vi "Lifetime at UC Intersection (gated).vi"(8 "Error In":errorcluster, 11 "Data for Pseudo UC Intersections":T1={"Linear Coefficients"={"u"=0.0, "v"=0.0}, "Decay Definition"={"offset: t0"=0.0, "period: T"=0.0, "lifetime: tau"=0.0, "Incident Signal: I"=0.0, "Normalized Decays"=FALSE, "IRF Model"=enum."Dirac", "IRF Parameter 1"=0.0, "Poisson Signal"=FALSE}, "Gates Definitions"={"First Gate: t1"=0.0, "Gate Width: W"=0.0, "Gate Step: d"=0.0, "# Gates: G"=0.0, "Use Gate Center"=FALSE, "Frames/Image: F"=0, "Gates/Frame: L"=0, "Bits/Frame: q"=0, "Multiplicity: p"=0, "Gate Type"=enum."Square", "Gate Edge s"=4.0, "Gate Top Slope"=4.0, "Reversed Sawtooth?"=FALSE, "Computation"=FALSE, "User-defined Gate"={"X Array"=[], "Y Array"=[]}, "Tolerance"=50.0, "Integration"=enum."Item 0", "# Steps"=50.0, "Type of User-defined Function"=enum."Gate"}, "iw"=0.0+0.0i, "Phasor Calculation"=enum."Direct Sum"}) -> (0 "Error Out":errorcluster, 1 "Analytical Solution 1":dbl[unit], 3 "Analytical Solution 2":dbl[unit])   [LabVIEW 2019]
uses:
  Data for SEPL Intersections.ctl
  Decay Definiton.ctl
  IRF Model.ctl
  Gate Definitions.ctl
  Gate Type.ctl
  Graphs/XY Graph/XY Plot Data.ctl
  Phasor Calculation Type.ctl
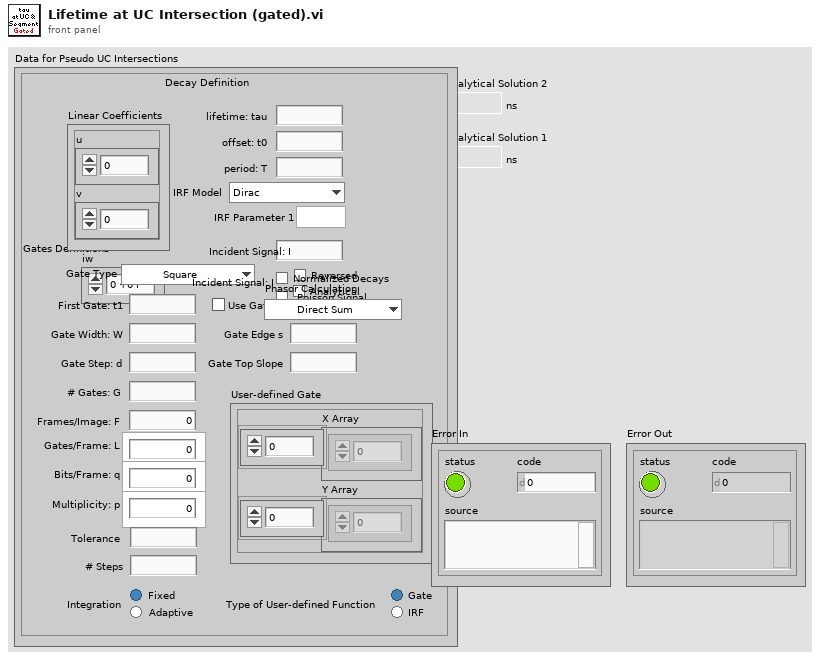
[diagram p1: front panel]
types:
  T1 = typedef "Data for SEPL Intersections.ctl" = cluster{"Linear Coefficients":cluster{"u":dbl, "v":dbl}, "Decay Definition":T2, "Gates Definitions":T4, "iw":cdb, "Phasor Calculation":T7}
  T2 = typedef "Decay Definiton.ctl" = cluster{"offset: t0":ext, "period: T":ext, "lifetime: tau":ext, "Incident Signal: I":ext, "Normalized Decays":bool, "IRF Model":T3, "IRF Parameter 1":ext, "Poisson Signal":bool}
  T3 = typedef "IRF Model.ctl" = enum16{"Dirac", "Exponential"}
  T4 = typedef "Gate Definitions.ctl" = cluster{"First Gate: t1":ext, "Gate Width: W":ext, "Gate Step: d":ext, "# Gates: G":ext, "Use Gate Center":bool, "Frames/Image: F":i32, "Gates/Frame: L":i32, "Bits/Frame: q":i32, "Multiplicity: p":i32, "Gate Type":T5, "Gate Edge s":ext, "Gate Top Slope":ext, "Reversed Sawtooth?":bool, "Computation":bool, "User-defined Gate":T6, "Tolerance":ext, "Integration":enum32{"Item 0", "Item 1"}, "# Steps":ext, "Type of User-defined Function":enum32{"Gate", "IRF"}}
  T5 = typedef "Gate Type.ctl" = enum16{"Square", "Finite Edge Square", "Finite Edge, Tilted Top Square", "Triangle", "Sawtooth", "User-defined"}
  T6 = typedef "XY Plot Data.ctl" = cluster{"X Array":dbl[], "Y Array":dbl[]}
  T7 = typedef "Phasor Calculation Type.ctl" = enum16{"Direct Sum", "Analytical Formula"}
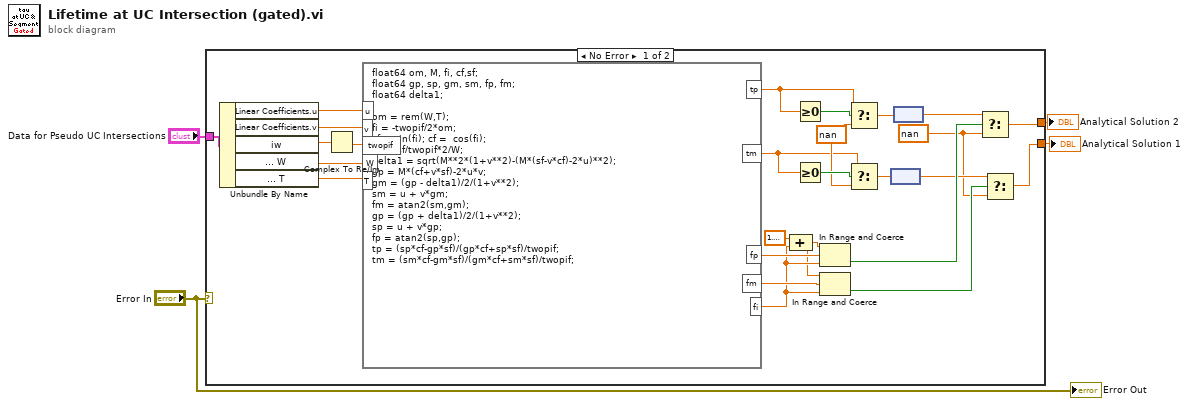
[diagram p0: block diagram]
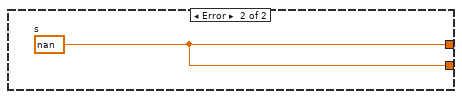
[diagram p2: hidden frame]
diagram:
  n1 = case shown="No Error" "Error In" {
    tunnel: "Data for Pseudo UC Intersections" -> [w30 _]
    tunnel: [w13 w31] -> w3
    tunnel: [w19 w31] -> w2
    frame No Error {
      w6 = nan ("f")
      w12 = dbl[unit] nan ("f")
      n2 = Unbundle By Name(w30) -> ("Linear Coefficients.u"=w29:dbl, "Linear Coefficients.v"=w28:dbl, "iw"=w27:cdb, "Gates Definitions.Gate Width: W"=w25:ext, "Decay Definition.period: T"=w24:ext)
      n3 = Complex To Re/Im(x + iy=w27) -> (y=w26:dbl)  [unwired: 1 out]
      n4 = formula code="float64 om, M, fi, cf,sf;\nfloat64 gp, sp, gm, sm, fp, fm;\nfloat64 delta1;\n\nom = rem(W,T);\nfi = -twopif/2*om;\nsf = sin(fi); cf =  cos(fi);\nM = -sf/twopif*2/W;\ndelta1 = sqrt(M**2*(1+v**2)-(M*(sf-v*cf)-2*u)**2);\ngp = M*(cf+v*sf)-2*u*v;\ngm = (gp - delta1)/2/(1+v**2);\nsm = u + v*gm;\nfm = atan2(sm,gm);\ngp = (gp + delta1)/2/(1+v**2);\nsp = u + v*gp;\nfp = atan2(sp,gp); \ntp = (sp*cf-gp*sf)/(gp*cf+sp*sf)/twopif;\ntm = (sm*cf-gm*sf)/(gm*cf+sm*sf)/twopif;"("u"=w29, "v"=w28, "twopif"=w26, "W"=w25, "T"=w24) -> ("tm"=w5:dbl, "tp"=w10:dbl, "fp"=w23:dbl, "fm"=w18:dbl, "fi"=w17:dbl)
      n5 = Compound Arithmetic op=ADD(1.5707963267948966, w17) -> (w16:dbl)
      n6 = Greater Or Equal To 0?(x=w10) -> (x >= 0?=w11:bool)
      n7 = Greater Or Equal To 0?(x=w5) -> (x >= 0?=w8:bool)
      n8 = In Range and Coerce(upper limit=w16, x=w23, lower limit=w17) -> (In Range?=w21:bool)  [unwired: 1 out]
      n9 = In Range and Coerce(upper limit=w16, x=w18, lower limit=w17) -> (In Range?=w15:bool)  [unwired: 1 out]
      n10 = Select(t=w10, s=w11, f=w6) -> (s? t:f=w9:dbl)
      n11 = Select(t=w5, s=w8, f=w6) -> (s? t:f=w7:dbl)
      n12 = node(w7) -> (w14:dbl[unit])
      n13 = node(w9) -> (w20:dbl[unit])
      n14 = Select(t=w20, s=w21, f=w12) -> (s? t:f=w19:dbl[unit])
      n15 = Select(t=w14, s=w15, f=w12) -> (s? t:f=w13:dbl[unit])
    }
    frame Error {
      w31 = dbl[unit] nan  # s
    }
  }
  "Analytical Solution 1" <- w3
  "Analytical Solution 2" <- w2
  "Error Out" <- "Error In"
